vi "delete.vi"(8 "error in (no error)":errorcluster, 11 "path":string) -> (0 "error out":errorcluster)   [LabVIEW 2015, in "lv-dropbox.lvlib" / "v2.lvlib"]
uses:
  v2.lvlib
  <vilib>/httpClient/POSTBuffer.vi
  <vilib>/httpClient/LabVIEWHTTPClient.lvlib
  lv-dropbox.lvlib
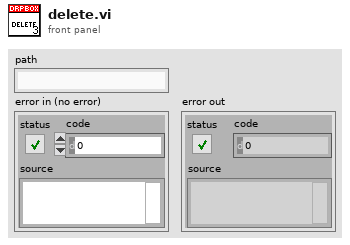
[diagram p1: front panel]
types:
  T1 = cluster{".tag":string, "name":string, "path_lower":string, "id":string, "client_modified":string, "server_modified":string, "rev":string, "size":u64}
  T2 = typedef "LabVIEWHTTPClient.lvlib/ClientHandle.ctl" = refnum<k1>
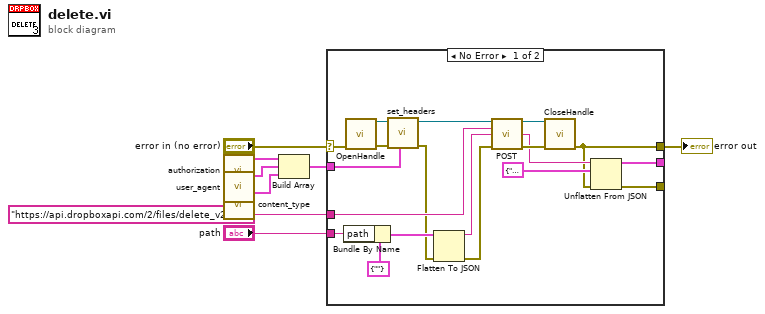
[diagram p0: block diagram]
diagram:
  n1 = call "authorization.vi"() -> ("header"=w5:cluster{"header":string, "value":string})  [unwired: 11 in]
  n2 = call "user_agent.vi"() -> ("header"=w4:cluster{"header":string, "value":string})  [unwired: 11 in]
  n3 = call "content_type.vi"() -> ("header"=w6:cluster{"header":string, "value":string})  [unwired: 11 in]
  n4 = Build Array(w5, w4, w6) -> (w1:cluster{"header":string, "value":string}[])
  n5 = case shown="No Error" "error in (no error)" {
    selector: "error in (no error)" -> [w19 w28]
    tunnel: [w10 w28] -> w7
    tunnel: "path" -> [w22 _]
    tunnel: "https://api.dropboxapi.com/2/files/delete_v2" ("url") -> [w16 _]
    tunnel: w1 -> [w15 _]
    tunnel: [w11 _] -> _
    tunnel: [w9 _] -> _
    frame No Error {
      n6 = Bundle By Name(cluster=cluster{"path":string} {"path"=""}, "path"=w22) -> (w23:cluster{"path":string})
      n7 = call <vilib>:"OpenHandle.vi"("error in (no error)"=w19) -> ("client handle out"=w18:T2, "error out"=w14:errorcluster)  [unwired: 13 in]
      n8 = call "set_headers.vi"("header_value []"=w15, "error in (no error)"=w14, "client_handle in"=w18) -> ("error out"=w13:errorcluster, "client_handle out"=w17:T2)  [unwired: 7 in]
      n9 = Flatten To JSON(anything=w23, error in (no error)=w13) -> (JSON string=w21:string, 11:w12:errorcluster)  [unwired: 1 in]
      n10 = call-poly <vilib>:"POST.vi"("client handle"=w17, "url"=w16, "buffer"=w21, "error in (no error)"=w12) -> ("client handle out"=w26:T2, "body"=w25:string, "error out"=w27:errorcluster)  [unwired: 8 in, 1 out]
      n11 = call <vilib>:"CloseHandle.vi"("client handle"=w26, "error in (no error)"=w27) -> ("error out"=w10:errorcluster)  [unwired: 13 in]
      n12 = Unflatten From JSON(JSON string=w25, type and defaults=T1 {".tag"="", "name"="", "path_lower"="", "id"="", "client_modified"="", "server_modified"="", "rev"="", "size"=0}, error in (no error)=w10) -> (value=w11:T1, error out=w9:errorcluster)  [unwired: 4 in]
    }
    frame Error {
    }
  }
  "error out" <- w7
